vi "pulse test.vi"() -> ()   [LabVIEW 2014]
uses:
  <userlib>/DAQNavi Polymorphic VI/create/DAQNavi Create Channel(CI-UpDown Count Value).vi
  <vilib>/DAQmx/write.llb/DAQmx Write (Analog DBL 1Chan 1Samp).vi
  <userlib>/DAQNavi Polymorphic VI/read/DAQNavi Read (Counter Count Value 1Chan 1Samp).vi
panel:
  out "position2":dbl
  out "position1":dbl
  out "电压2":dbl
  out "电压1":dbl
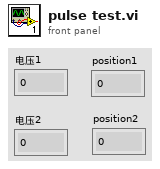
[diagram p1: front panel]
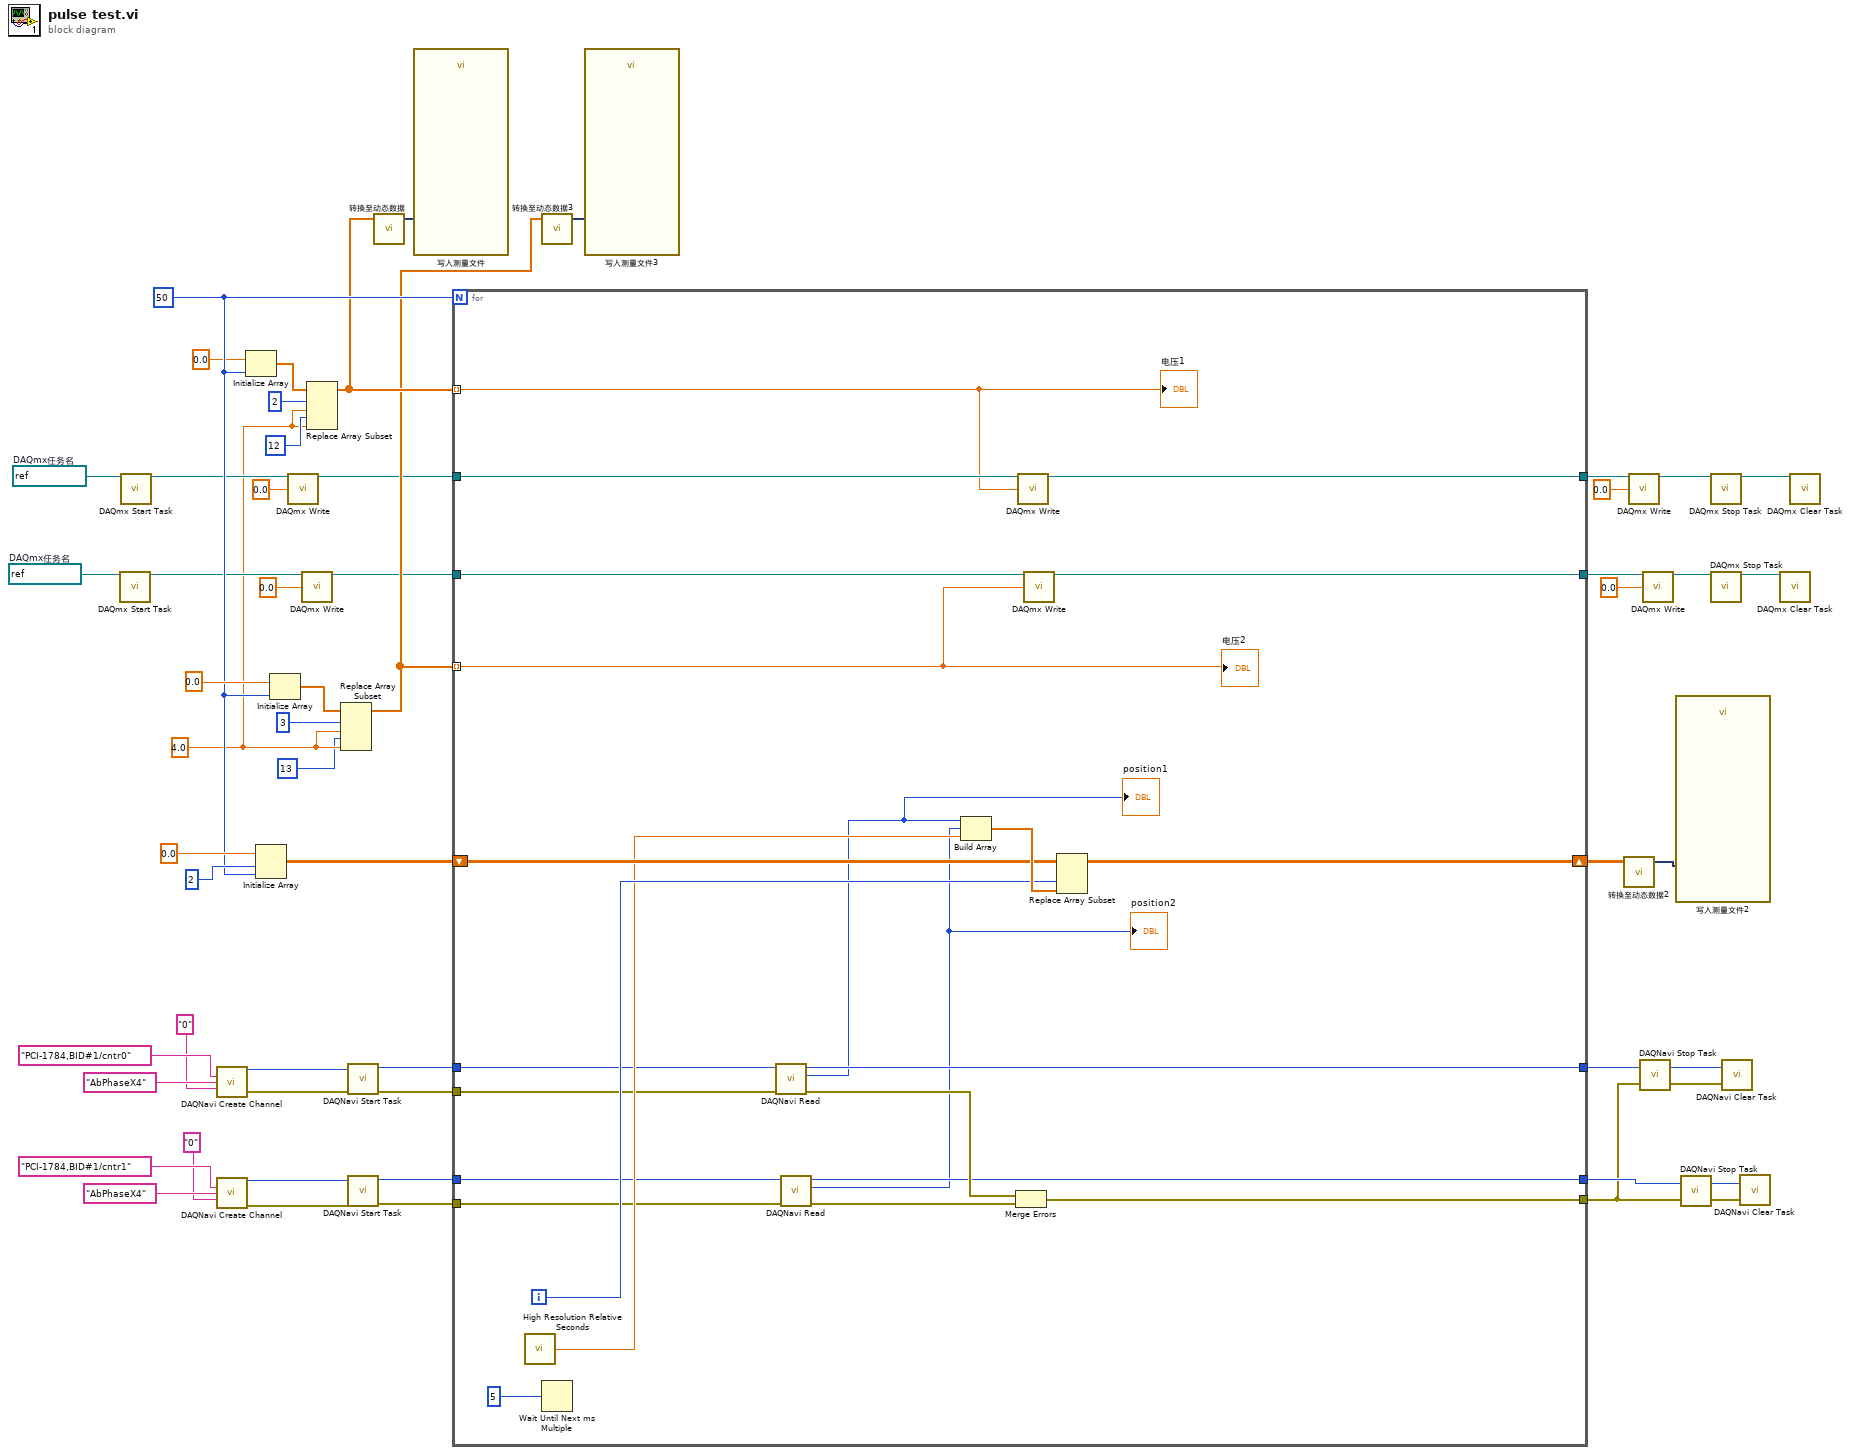
[diagram p0: block diagram]
diagram:
  w2 = 4.0
  w19 = 50
  w55 = refnum<k21> "Stage_Y"  # DAQmx任务名
  w56 = refnum<k21> "Stage_X"  # DAQmx任务名
  n1 = call <vilib>:"DAQmx Start Task.vi"("task/channels in"=w55) -> ("task out"=w7:refnum<k21>)  [unwired: 13 in, 1 out]
  n2 = call <vilib>:"DAQmx Start Task.vi"("task/channels in"=w56) -> ("task out"=w5:refnum<k21>)  [unwired: 13 in, 1 out]
  n3 = call-poly <userlib>:"DAQNavi Create Channel.vi"("physical channels"="PCI-1784,BID#1/cntr0" ("Image Name"), "signal counting type"="AbPhaseX4" ("Image Name"), "initial value"="0" ("Image Name")) -> ("task out"=w37:i32, "error out"=w36:errorcluster)  [unwired: 11 in]
  n4 = call-poly <userlib>:"DAQNavi Create Channel.vi"("physical channels"="PCI-1784,BID#1/cntr1" ("Image Name"), "signal counting type"="AbPhaseX4" ("Image Name"), "initial value"="0" ("Image Name")) -> ("task out"=w35:i32, "error out"=w34:errorcluster)  [unwired: 11 in]
  n5 = Initialize Array(0.0, w19) -> (w17:dbl[])
  n6 = Initialize Array(0.0, 2, w19) -> (w44:dbl[][])
  n7 = Initialize Array(0.0, w19) -> (w11:dbl[])
  n8 = call-poly <vilib>:"DAQmx Write.vi"("task/channels in"=w5, "data"=0.0) -> ("task out"=w4:refnum<k21>)  [unwired: 11 in, 2 out]
  n9 = call-poly <vilib>:"DAQmx Write.vi"("task/channels in"=w7, "data"=0.0) -> ("task out"=w6:refnum<k21>)  [unwired: 11 in, 2 out]
  n10 = Replace Array Subset(array=w17, new element #1=w2, index #1=2, new element #2=w2, index #2=12) -> (w15:dbl[])
  n11 = Replace Array Subset(array=w11, new element #1=w2, index #1=3, new element #2=w2, index #2=13) -> (w10:dbl[])
  n12 = call <userlib>:"DAQNavi Start Task.vi"("error in (no error)"=w36, "task in"=w37) -> ("error out"=w31:errorcluster, "task out"=w30:i32)  [unwired: 8 in]
  n13 = call <userlib>:"DAQNavi Start Task.vi"("error in (no error)"=w34, "task in"=w35) -> ("error out"=w28:errorcluster, "task out"=w29:i32)  [unwired: 8 in]
  n14 = call "转换至动态数据"("Array"=w15) -> ("Dynamic Data Type"=w14:dynamicdata)  [unwired: 3 in]
  n15 = call "写入测量文件"("Signals"=w14) -> ()  [unwired: 16 in, 3 out]
  n16 = for {
    N: w19 -> [_]
    tunnel: w4 -> [w79]
    tunnel: w6 -> [w78]
    tunnel: [w77] -> w48
    tunnel: [w76] -> w47
    shift-right: [w72] -> w43
    shift-left: w44 -> [w73]
    tunnel: w10 -> [w70] mode=indexing
    tunnel: w15 -> [w69] mode=indexing
    tunnel: w31 -> [w65]
    tunnel: w30 -> [w64]
    tunnel: w29 -> [w63]
    tunnel: w28 -> [w62]
    tunnel: [w61] -> w23
    tunnel: [w60] -> w22
    tunnel: [w59] -> w21
    i -> [w71]
    n17 = call <vilib>:"High Resolution Relative Seconds.vi"() -> ("relative seconds"=w68:dbl)
    n18 = Wait Until Next ms Multiple(millisecond multiple=5) -> ()  [unwired: 1 out]
    n19 = call-poly <userlib>:"DAQNavi Read.vi"("error in (no error)"=w65, "task in"=w64) -> ("error out"=w66:errorcluster, "data"=w57:i32, "task out"=w61:i32)  [unwired: 7 in]
    "position1" <- w57
    n20 = call-poly <userlib>:"DAQNavi Read.vi"("error in (no error)"=w62, "task in"=w63) -> ("error out"=w67:errorcluster, "data"=w58:i32, "task out"=w60:i32)  [unwired: 7 in]
    "position2" <- w58
    n21 = Build Array(w57, w58, w68) -> (w74:dbl[])
    n22 = Merge Errors(w66, w67) -> (w59:errorcluster)
    n23 = call-poly <vilib>:"DAQmx Write.vi"("task/channels in"=w79, "data"=w69) -> ("task out"=w77:refnum<k21>)  [unwired: 11 in, 2 out]
    n24 = call-poly <vilib>:"DAQmx Write.vi"("task/channels in"=w78, "data"=w70) -> ("task out"=w76:refnum<k21>)  [unwired: 11 in, 2 out]
    n25 = Replace Array Subset(array=w73, new element=w74, index (col)=w71) -> (w72:dbl[][])  [unwired: 1 in]
    "电压1" <- w69
    "电压2" <- w70
  }
  n26 = call "转换至动态数据3"("Array"=w10) -> ("Dynamic Data Type"=w13:dynamicdata)  [unwired: 3 in]
  n27 = call "写入测量文件3"("Signals"=w13) -> ()  [unwired: 16 in, 3 out]
  n28 = call "转换至动态数据2"("2D Array"=w43) -> ("Dynamic Data Type"=w46:dynamicdata)  [unwired: 3 in]
  n29 = call-poly <vilib>:"DAQmx Write.vi"("task/channels in"=w48, "data"=0.0) -> ("task out"=w54:refnum<k21>)  [unwired: 11 in, 2 out]
  n30 = call <userlib>:"DAQNavi Stop Task.vi"("error in (no error)"=w21, "task in"=w23) -> ("error out"=w26:errorcluster, "task out"=w27:i32)
  n31 = call-poly <vilib>:"DAQmx Write.vi"("task/channels in"=w47, "data"=0.0) -> ("task out"=w52:refnum<k21>)  [unwired: 11 in, 2 out]
  n32 = call "写入测量文件2"("Signals"=w46) -> ()  [unwired: 16 in, 3 out]
  n33 = call <userlib>:"DAQNavi Stop Task.vi"("error in (no error)"=w21, "task in"=w22) -> ("error out"=w24:errorcluster, "task out"=w25:i32)
  n34 = call <vilib>:"DAQmx Stop Task.vi"("task/channels in"=w54) -> ("task out"=w50:refnum<k21>)  [unwired: 13 in, 1 out]
  n35 = call <vilib>:"DAQmx Stop Task.vi"("task/channels in"=w52) -> ("task out"=w49:refnum<k21>)  [unwired: 13 in, 1 out]
  n36 = call <userlib>:"DAQNavi Clear Task.vi"("error in (no error)"=w26, "task in"=w27) -> ()  [unwired: 1 in, 1 out]
  n37 = call <userlib>:"DAQNavi Clear Task.vi"("error in (no error)"=w24, "task in"=w25) -> ()  [unwired: 1 in, 1 out]
  n38 = call <vilib>:"DAQmx Clear Task.vi"("task in"=w49) -> ()  [unwired: 14 in, 1 out]
  n39 = call <vilib>:"DAQmx Clear Task.vi"("task in"=w50) -> ()  [unwired: 14 in, 1 out]
